vi "更新全局变量.vi"() -> ()   [LabVIEW 2016, in "数据传输系统-05.lvlib" / "update.lvlib"]
uses:
  update.lvlib
  http client class/http client.lvclass
  WebDAV client/WebDAV client.lvclass
panel:
  in  "WebDAV client 输入":refnum<class "WebDAV client.lvclass">
  in  "http client 输入":refnum<class "http client.lvclass">
  out "文件大小":i64
  out "已下载大小":i64
  out "滑动杆":dbl(slide) scale=0.0..100.0
  out "command":string caption="命令"
  out "last status string":string caption="最近状态字符串"
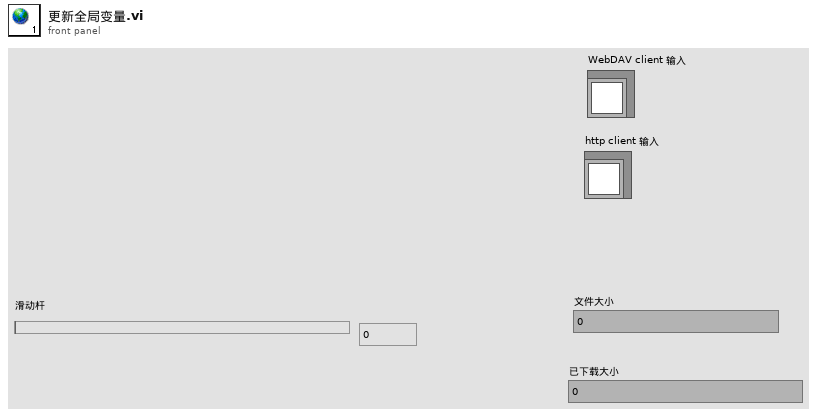
[diagram p1: front panel]
diagram:
